vi "BRig_FPGA_v3,93__PortC.vi"() -> ()   [LabVIEW 2014]
uses:
  <vilib>/rvi/Emulation/niFpgaGetClockAttributes.vi
  <vilib>/rvi/Emulation/niFpgaSctlEmulationGetInTimedLoop.vi
  <vilib>/rvi/Emulation/niFpgaEmulationReportErrorSimple.vi
  <vilib>/rvi/eio/common/nirviEmuTemplateMethod_errors.vi
  <vilib>/rvi/Emulation/niFpgaCriticalErrorInLSC.vi
  <vilib>/eio/EIONode/EIONode.xnode
panel:
  out "fpga_solenoid_R":bool
  out "fpga_solenoid_L":bool
  out "fpga_laser2":bool
  out "fpga_laser1":bool
  in  "L2Led_ON":bool
  in  "L1Led_ON":bool
  in  "Rising(F)_or_Falling(T)":bool
  in  "Solenoid_trig_R":bool
  in  "Solenoid_trig_L":bool
  in  "Solenoid_nTotal_R":u32=100
  in  "Solenoid_nTotal_L":u32=100
  in  "L2Led_Baseline":bool
  in  "L1Led_Baseline":bool
  in  "CueLed_Baseline":bool
  in  "I_allReward":bool
  in  "AnaOut_1":i16
  in  "CueLed_Event":bool
  in  "CueLed_nValley":u32=100
  in  "CueLed_nPeak":u32=100
  in  "LC_Event_l2":bool
  in  "LC_Laser_l2":bool
  in  "LC_nShutter_l2":u32=100
  in  "LC_nValley_l2":u32=100
  in  "LC_nPeak_l2":u32=100
  in  "LR_wrong_nDelay_l2":u32
  in  "LR_reward_nDelay_l2":u32
  in  "LR_wrong_nTotal_l2":u32=100
  in  "LR_reward_nTotal_l2":u32=100
  in  "LR_wrong_laser_l2":bool
  in  "LR_wrong_Event_l2":bool
  in  "LR_reward_Laser_l2":bool
  in  "LR_reward_Event_l2":bool
  out "AnaIn_1":i16
  out "AnaIn_0":i16
  out "timeTrial_count":u32
  in  "timeTrial_trig":bool
  in  "k1__counter_per_ms":u16=100 min=100 max=40000 step=1
  in  "LC_nShutter_l1":u32=100
  in  "AnaOut_0":i16
  in  "LC_nValley_l1":u32=100
  in  "LC_nPeak_l1":u32=100
  in  "LC_Event_l1":bool
  in  "LR_wrong_nTotal_l1":u32=100
  in  "LR_wrong_nDelay_l1":u32
  in  "LR_reward_nTotal_l1":u32=100
  in  "LR_reward_nDelay_l1":u32
  in  "LR_reward_Event_l1":bool
  in  "LR_wrong_Event_l1":bool
  out "SelectWrong":bool
  out "SelectReward":bool
  in  "LR_wrong_Laser_l1":bool
  in  "LR_reward_Laser_l1":bool
  in  "Left(F)_or_Right(T)":bool
  in  "ignoreWrong":bool
  in  "SelectionState":bool
  in  "LC_Laser_l1":bool
  in  "FPGA_Stop":bool
  in  "audioTrigger_L":bool
  in  "audioTrigger_R":bool
  in  "audioFreq_L_kHz":u8=14 min=1 max=14 step=1
  in  "audioAmp_L":u16=1 min=1 max=32767 step=1
  in  "audioFreq_R_kHz":u8=14 min=1 max=14 step=1
  in  "audioAmp_R":u16=1 min=1 max=32767 step=1
  in  "A3_SL":bool
  in  "A1_SR":bool
  in  "Counts_Reset":bool
  out "A4_LickR":u32
  out "A2_LickL":u32
  in  "A6_Act":bool
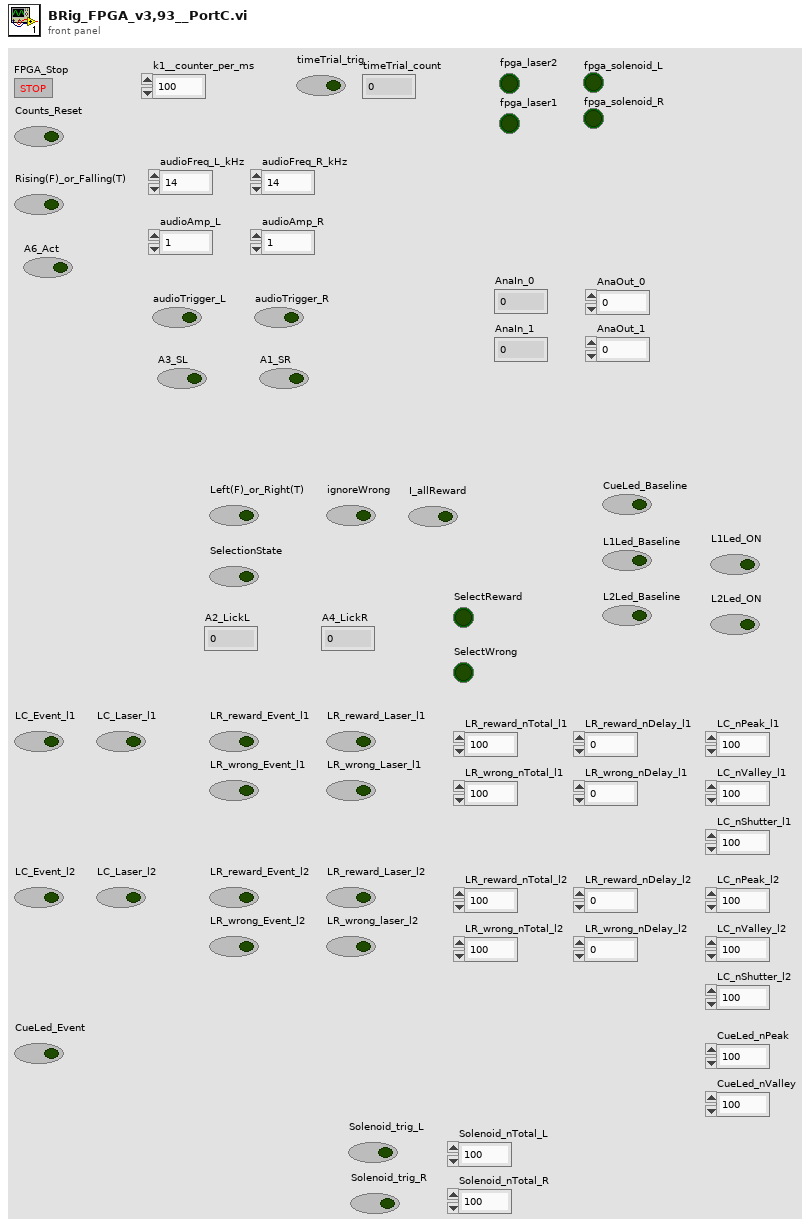
[diagram p1: front panel]
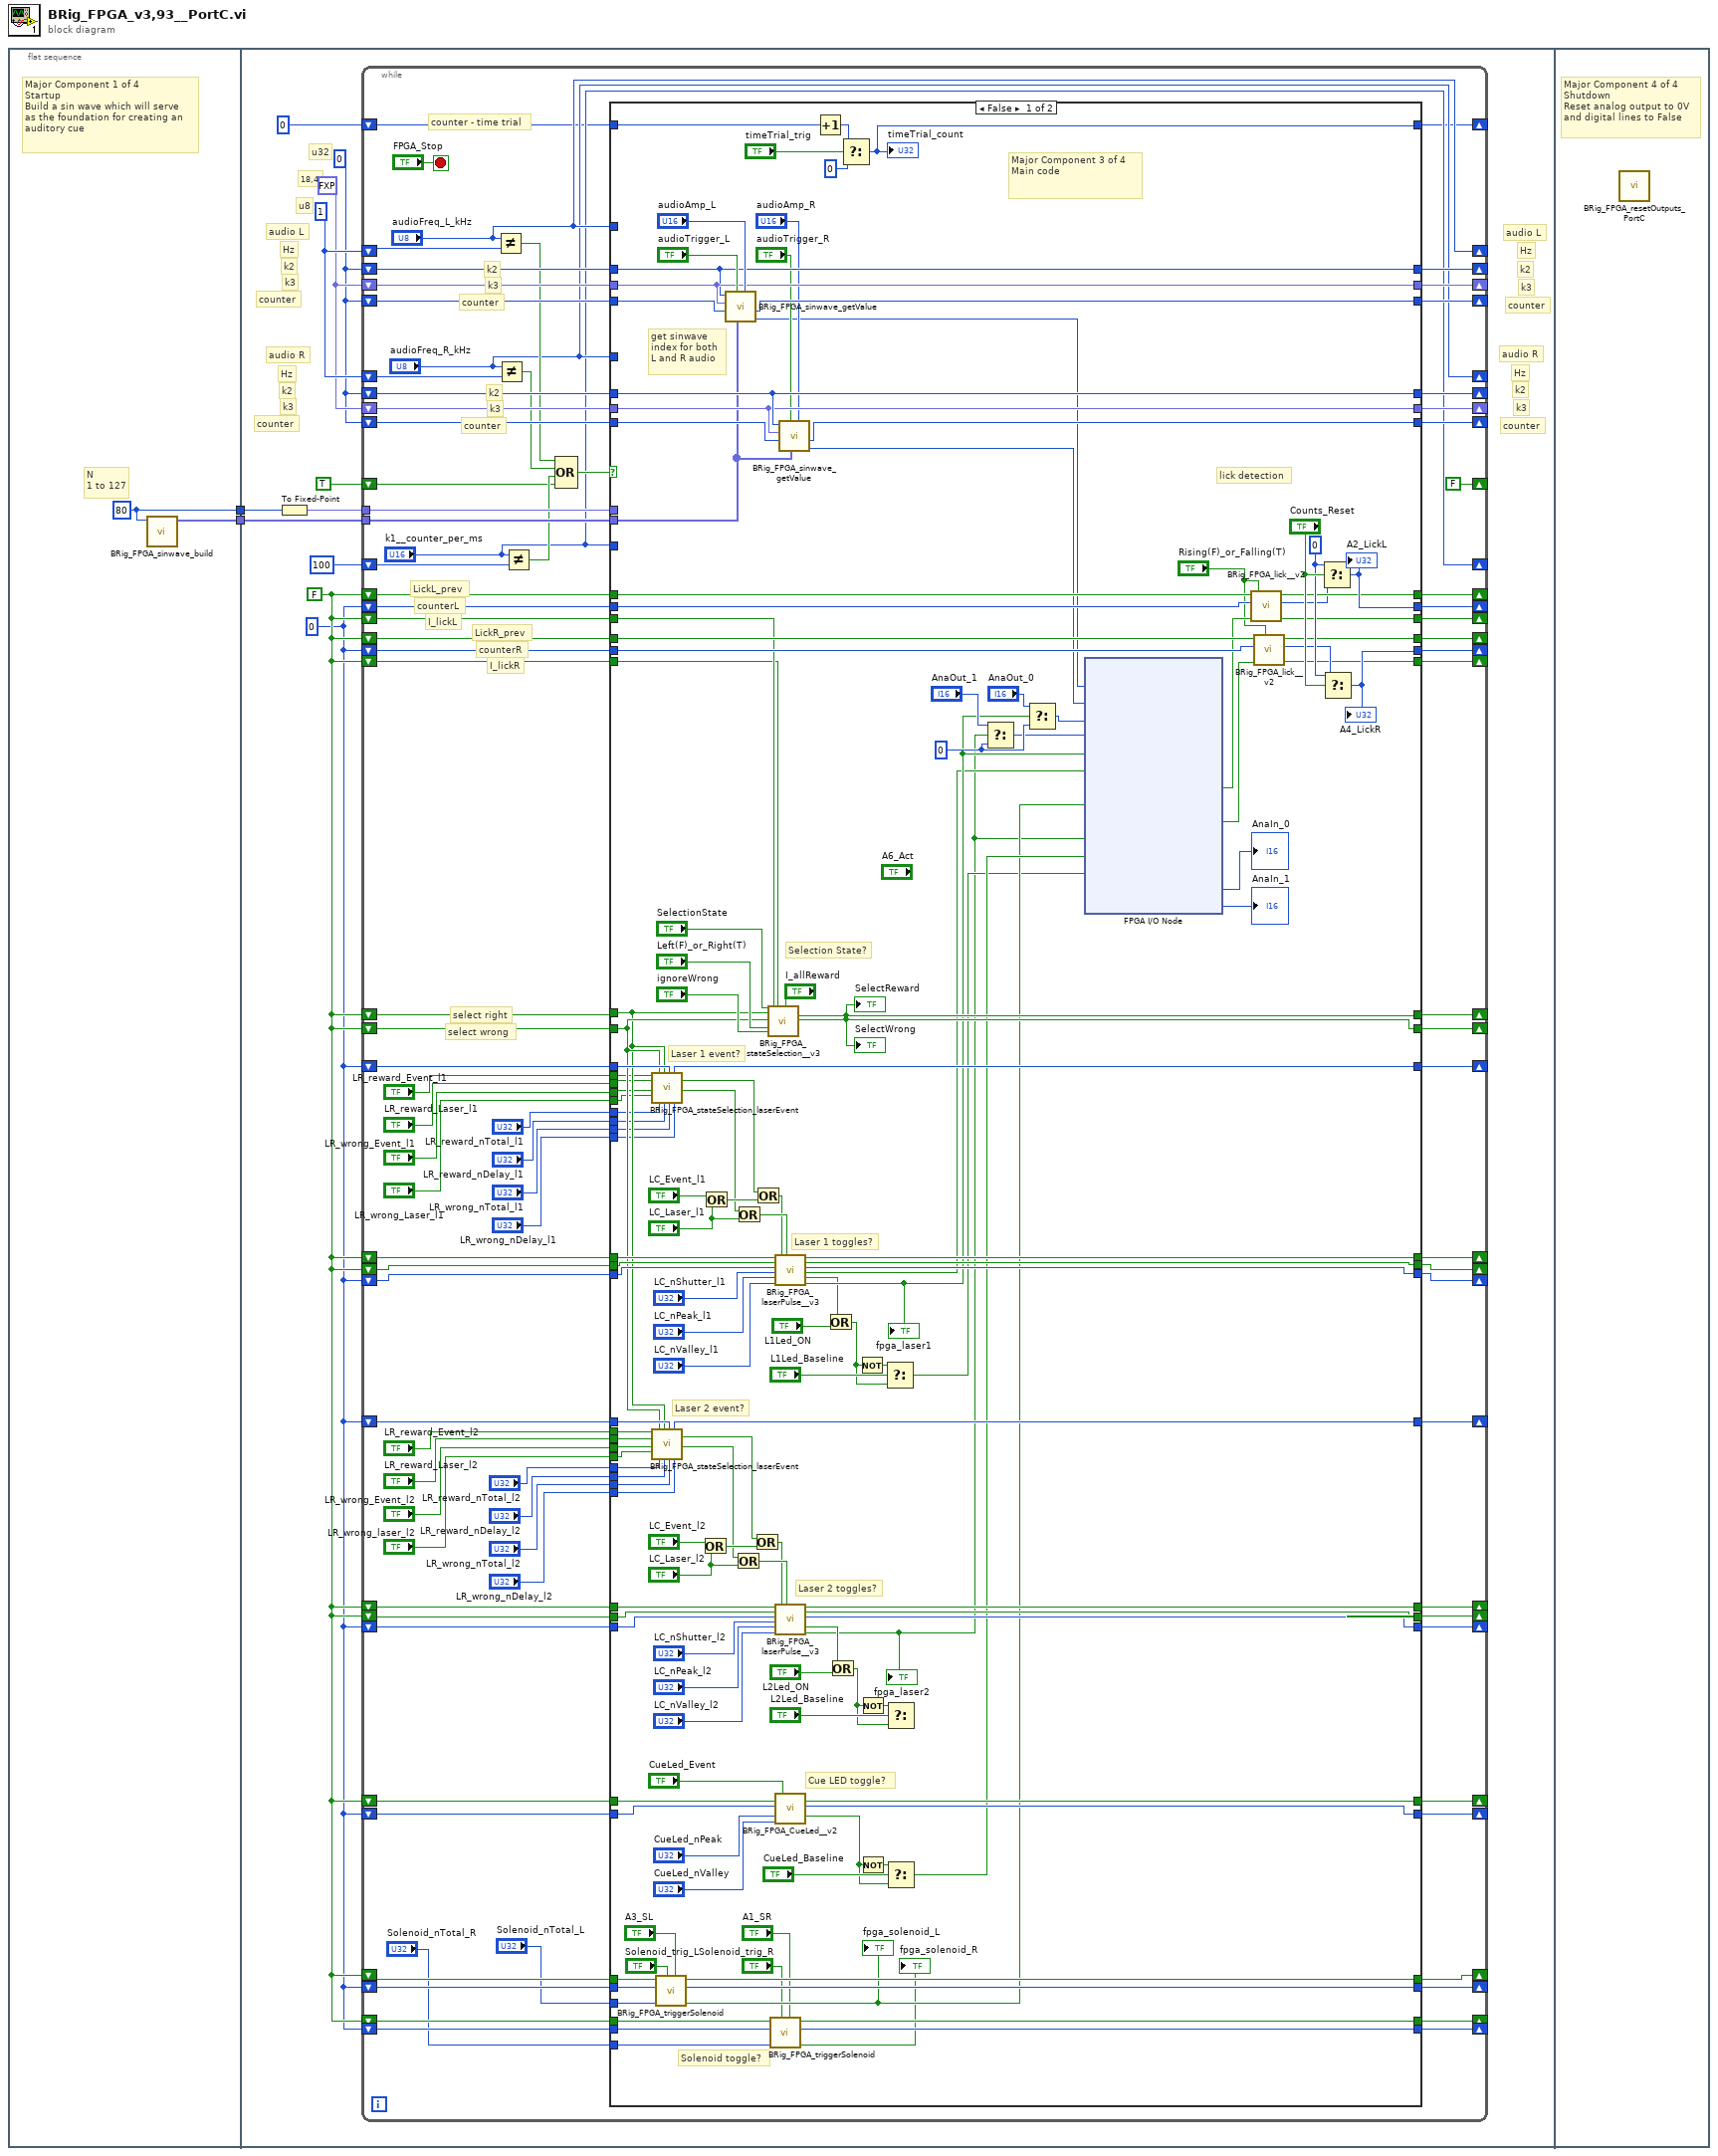
[diagram p0: block diagram]
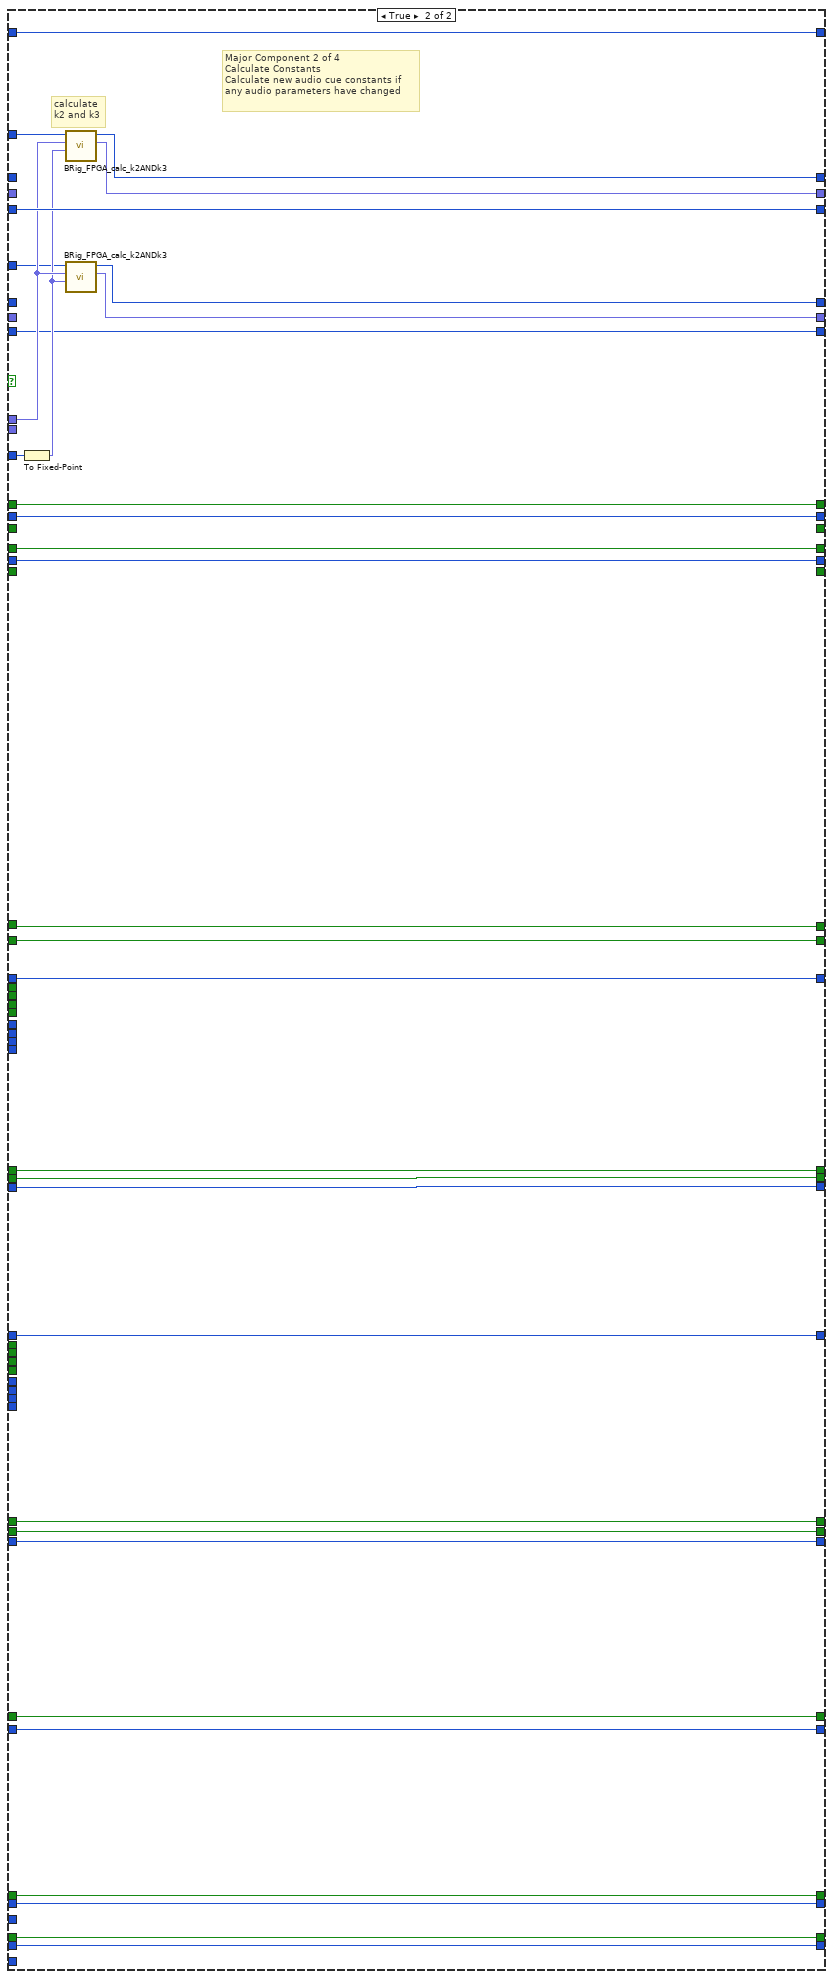
[diagram p2: hidden frame]
diagram:
  n1 = flat-sequence {
    tunnel: [w4] -> w2
    tunnel: [w3] -> w1
    tunnel: w2 -> [w15]
    tunnel: w1 -> [w14]
    frame #0 {
      w3 = 80 ("dimension size")
      # "Major Component 1 of 4\nStartup\nBuild a sin wave which will serve\nas the foundation for creating an\nauditory cue"
      # "N\n1 to 127"
      n2 = call "BRig_FPGA_sinwave_build.vi"("input_Npts"=w3) -> ("output_array_sin"=w4:fxp<+/-,16,2>[])  [unwired: 10 in]
    }
    frame #1 {
      w5 = u32 0
      w6 = FALSE
      w10 = u32 0
      w11 = fxp<+,18,4> 0.0
      w12 = u8 1
      # "counter"
      # "k3"
      # "k2"
      # "counter"
      # "k3"
      # "k2"
      # "counter"
      # "counter"
      # "u32"
      # "k3"
      # "k2"
      # "k3"
      # "18,4"
      # "u8"
      # "Hz"
      # "Hz"
      # "audio R"
      # "audio L"
      # "Hz"
      # "k2"
      # "Hz"
      # "audio R"
      # "audio L"
      n3 = To Fixed-Point(number=w14) -> (fixed-point=w13:fxp<+,7,7>)  [unwired: 1 in]
      n4 = while {
        shift-right: ["audioFreq_L_kHz"] -> _
        shift-left: w12 -> [w106]
        shift-right: [w100] -> _
        shift-left: w10 -> [w104]
        shift-right: ["audioFreq_R_kHz"] -> _
        shift-left: w12 -> [w96]
        tunnel: w15 -> [w103]
        tunnel: w13 -> [w102]
        shift-right: [w99] -> _
        shift-left: w11 -> [w101]
        shift-right: [w97] -> _
        shift-left: w10 -> [w98]
        shift-right: [w94] -> _
        shift-left: w10 -> [w95]
        shift-right: [w92] -> _
        shift-left: w11 -> [w93]
        shift-right: [w90] -> _
        shift-left: w10 -> [w91]
        shift-right: ["k1__counter_per_ms"] -> _
        shift-left: u16 100 ("y") -> [w89]
        shift-right: [FALSE] -> _
        shift-left: TRUE -> [w84]
        shift-right: [w77] -> _
        shift-left: w6 -> [w79]
        shift-right: [w76] -> _
        shift-left: w6 -> [w78]
        shift-right: [w74] -> _
        shift-left: w5 -> [w75]
        shift-right: [w72] -> _
        shift-left: w5 -> [w73]
        shift-right: [w69] -> _
        shift-left: w6 -> [w71]
        shift-right: [w68] -> _
        shift-left: w6 -> [w70]
        shift-right: [w66] -> _
        shift-left: w6 -> [w67]
        shift-right: [w64] -> _
        shift-left: w6 -> [w65]
        shift-right: [w62] -> _
        shift-left: u32 0 -> [w63]
        shift-right: [w60] -> _
        shift-left: w5 -> [w61]
        shift-right: [w59] -> _
        shift-left: w6 -> [w56]
        shift-right: [w58] -> _
        shift-left: w6 -> [w55]
        shift-right: [w57] -> _
        shift-left: w5 -> [w54]
        shift-right: [w52] -> _
        shift-left: w5 -> [w53]
        shift-right: [w51] -> _
        shift-left: w6 -> [w48]
        shift-right: [w50] -> _
        shift-left: w6 -> [w47]
        shift-right: [w49] -> _
        shift-left: w5 -> [w46]
        shift-right: [w45] -> _
        shift-left: w6 -> [w43]
        shift-right: [w44] -> _
        shift-left: w5 -> [w42]
        shift-right: [w24] -> _
        shift-left: w5 -> [w25]
        shift-right: [w21] -> _
        shift-left: w6 -> [w23]
        shift-right: [w18] -> _
        shift-left: w6 -> [w20]
        shift-right: [w17] -> _
        shift-left: w5 -> [w19]
        stop <- "FPGA_Stop" stop-if-true
        # "counter"
        # "k3"
        # "k2"
        # "counter"
        # "k3"
        # "k2"
        # "counter - time trial"
        # "I_lickR"
        # "counterR"
        # "LickR_prev"
        # "I_lickL"
        # "counterL"
        # "LickL_prev"
        # "select wrong"
        # "select right"
        n5 = Not Equal?(x="audioFreq_L_kHz", y=w106) -> (x != y?=w88:bool)
        n6 = Not Equal?(x="audioFreq_R_kHz", y=w96) -> (x != y?=w87:bool)
        n7 = Not Equal?(x="k1__counter_per_ms", y=w89) -> (x != y?=w85:bool)
        n8 = Compound Arithmetic op=OR(w88, w87, w85, w84) -> (w86:bool)
        n9 = case shown="False" w86 {
          tunnel: w104 -> [w238 _]
          tunnel: "audioFreq_L_kHz" -> [_ w284]
          tunnel: w103 -> [w231 _]
          tunnel: w102 -> [_ w280]
          tunnel: "k1__counter_per_ms" -> [_ w285]
          tunnel: w101 -> [w239 _]
          tunnel: [w238 w283] -> w100
          tunnel: [w239 w282] -> w99
          tunnel: w98 -> [w243 w281]
          tunnel: [w240 w281] -> w97
          tunnel: w95 -> [w235 _]
          tunnel: [w235 w276] -> w94
          tunnel: w93 -> [w234 _]
          tunnel: [w234 w277] -> w92
          tunnel: w91 -> [w237 w275]
          tunnel: "audioFreq_R_kHz" -> [_ w278]
          tunnel: [w236 w275] -> w90
          tunnel: w79 -> [w226 w274]
          tunnel: w78 -> [w225 w273]
          tunnel: [w230 w274] -> w77
          tunnel: [w223 w273] -> w76
          tunnel: w75 -> [w227 w272]
          tunnel: [w253 w272] -> w74
          tunnel: w73 -> [w224 w271]
          tunnel: [w250 w271] -> w72
          tunnel: w71 -> [w177 w270]
          tunnel: w70 -> [w178 w269]
          tunnel: [w197 w270] -> w69
          tunnel: [w246 w269] -> w68
          tunnel: [w216 w266] -> w59
          tunnel: [w217 w265] -> w58
          tunnel: [w218 w264] -> w57
          tunnel: w67 -> [w220 _]
          tunnel: [w229 _] -> w66
          tunnel: w65 -> [w219 _]
          tunnel: [w221 _] -> w64
          tunnel: w63 -> [w208 w268]
          tunnel: [w205 w268] -> w62
          tunnel: w61 -> [w196 w267]
          tunnel: [w195 w267] -> w60
          tunnel: w56 -> [w194 w266]
          tunnel: w55 -> [w193 w265]
          tunnel: w54 -> [w192 w264]
          tunnel: w53 -> [w180 w263]
          tunnel: [w179 w263] -> w52
          tunnel: [w175 w262] -> w51
          tunnel: [w174 w261] -> w50
          tunnel: [w173 w260] -> w49
          tunnel: w48 -> [w172 w262]
          tunnel: w47 -> [w171 w261]
          tunnel: w46 -> [w170 w260]
          tunnel: [w167 w259] -> w45
          tunnel: [w166 w258] -> w44
          tunnel: w43 -> [w165 w259]
          tunnel: w42 -> [w164 w258]
          tunnel: "LR_reward_Event_l1" -> [w148 _]
          tunnel: "LR_reward_Laser_l1" -> [w147 _]
          tunnel: "LR_wrong_Event_l1" -> [w146 _]
          tunnel: "LR_wrong_Laser_l1" -> [w145 _]
          tunnel: "LR_reward_nTotal_l1" -> [w144 _]
          tunnel: "LR_reward_nDelay_l1" -> [w143 _]
          tunnel: "LR_wrong_nTotal_l1" -> [w142 _]
          tunnel: "LR_wrong_nDelay_l1" -> [w141 _]
          tunnel: "LR_reward_Event_l2" -> [w140 _]
          tunnel: "LR_reward_Laser_l2" -> [w139 _]
          tunnel: "LR_wrong_Event_l2" -> [w138 _]
          tunnel: "LR_wrong_laser_l2" -> [w137 _]
          tunnel: "LR_reward_nTotal_l2" -> [w136 _]
          tunnel: "LR_reward_nDelay_l2" -> [w135 _]
          tunnel: "LR_wrong_nTotal_l2" -> [w134 _]
          tunnel: "LR_wrong_nDelay_l2" -> [w133 _]
          tunnel: w25 -> [w132 w257]
          tunnel: [w127 w257] -> w24
          tunnel: w23 -> [w131 w256]
          tunnel: "Solenoid_nTotal_L" -> [w130 _]
          tunnel: [w126 w256] -> w21
          tunnel: w20 -> [w122 w255]
          tunnel: w19 -> [w121 w254]
          tunnel: [w120 w255] -> w18
          tunnel: [w119 w254] -> w17
          tunnel: "Solenoid_nTotal_R" -> [w118 _]
          frame False {
            w161 = i16 0 ("f")
            w251 = u32 0 ("t")
            # "Solenoid toggle?"
            # "Cue LED toggle?"
            # "Laser 2 toggles?"
            # "Laser 2 event?"
            # "Laser 1 toggles?"
            # "Selection State?"
            # "Laser 1 event?"
            # "Major Component 3 of 4\nMain code"
            # "get sinwave\nindex for both\nL and R audio"
            # "lick detection"
            n10 = call "BRig_FPGA_stateSelection_laserEvent.vi"("I_LR_reward"=w148, "I_LR_reward_laser"=w147, "I_LR_wrong"=w146, "I_LR_wrong_laser"=w145, "I_selectWrong"=w178, "laser_reward_nTotal"=w144, "I_selectReward"=w177, "laser_reward_nDelay"=w143, "counter"=w196, "laser_wrong_nTotal"=w142, "laser_wrong_nDelay"=w141) -> ("output_counter"=w195:u32, "output_I_laserEvent"=w191:bool, "output_I_laserOn"=w190:bool)  [unwired: 6 in]
            n11 = call "BRig_FPGA_stateSelection_laserEvent.vi"("I_LR_reward"=w140, "I_LR_reward_laser"=w139, "I_LR_wrong"=w138, "I_LR_wrong_laser"=w137, "I_selectWrong"=w178, "laser_reward_nTotal"=w136, "I_selectReward"=w177, "laser_reward_nDelay"=w135, "counter"=w180, "laser_wrong_nTotal"=w134, "laser_wrong_nDelay"=w133) -> ("output_counter"=w179:u32, "output_I_laserEvent"=w176:bool, "output_I_laserOn"=w181:bool)  [unwired: 6 in]
            n12 = call "BRig_FPGA_triggerSolenoid.vi"("input_Solenoid_MTrig"="A3_SL", "input_Solenoid_trig"="Solenoid_trig_L", "input_threshold"=w130, "input_counter"=w132, "input_trig"=w131) -> ("output_Solenoid_OnOff"=w125:bool, "output_counter"=w127:u32, "output_trig"=w126:bool)  [unwired: 4 in]
            "fpga_solenoid_L" <- w125
            n13 = Or(x="LC_Event_l2", y="LC_Laser_l2") -> (x .or. y?=w185:bool)
            n14 = Or(x="LC_Event_l1", y="LC_Laser_l1") -> (x .or. y?=w212:bool)
            n15 = call "BRig_FPGA_sinwave_getValue.vi"("audioAmp"="audioAmp_L", "sinwave"=w231, "audioTrigger"="audioTrigger_L", "counter"=w243, "k3"=w239, "k2"=w238) -> ("output_audioValue"=w203:i16, "output_counter"=w240:u32)  [unwired: 4 in]
            n16 = Or(x=w181, y="LC_Laser_l2") -> (x .or. y?=w183:bool)
            n17 = Or(x=w190, y="LC_Laser_l1") -> (x .or. y?=w210:bool)
            n18 = Or(x=w176, y=w185) -> (x .or. y?=w182:bool)
            n19 = Or(x=w191, y=w212) -> (x .or. y?=w209:bool)
            n20 = call "BRig_FPGA_stateSelection__v3.vi"("I_selectionState"="SelectionState", "I_selectRight"=w177, "I_selectWrong"=w178, "I_Left(F)_or_Right(T)"="Left(F)_or_Right(T)", "I_ignoreWrong"="ignoreWrong", "I_lickL"=w220, "I_lickR"=w219, "I_allReward"="I_allReward") -> ("output__I_selectRight"=w197:bool, "output__I_selectWrong"=w246:bool)  [unwired: 18 in]
            "SelectWrong" <- w246
            "SelectReward" <- w197
            n21 = call "BRig_FPGA_triggerSolenoid.vi"("input_Solenoid_MTrig"="A1_SR", "input_Solenoid_trig"="Solenoid_trig_R", "input_threshold"=w118, "input_counter"=w121, "input_trig"=w122) -> ("output_Solenoid_OnOff"=→"fpga_solenoid_R":bool, "output_counter"=w119:u32, "output_trig"=w120:bool)  [unwired: 4 in]
            n22 = call "BRig_FPGA_laserPulse__v3.vi"("I_shutter"=w194, "I_peak"=w193, "count"=w192, "laser_Nshutter"="LC_nShutter_l1", "laser_Npeak"="LC_nPeak_l1", "laser_Nvalley"="LC_nValley_l1", "I_laserEvent"=w209, "I_laser"=w210) -> ("output_I_shutter"=w216:bool, "output_I_peak"=w217:bool, "output_count"=w218:u32, "output_shutter"=w109:bool, "output_led"=w114:bool, "output_laser"=w159:bool)  [unwired: 6 in]
            "fpga_laser1" <- w159
            n23 = call "BRig_FPGA_laserPulse__v3.vi"("I_shutter"=w172, "I_peak"=w171, "count"=w170, "laser_Nshutter"="LC_nShutter_l2", "laser_Npeak"="LC_nPeak_l2", "laser_Nvalley"="LC_nValley_l2", "I_laserEvent"=w182, "I_laser"=w183) -> ("output_I_shutter"=w175:bool, "output_I_peak"=w174:bool, "output_count"=w173:u32, "output_led"=w111:bool, "output_laser"=w108:bool)  [unwired: 6 in, 1 out]
            "fpga_laser2" <- w108
            n24 = call "BRig_FPGA_CueLed__v2.vi"("I_peak"=w165, "count"=w164, "laser_Npeak"="CueLed_nPeak", "laser_Nvalley"="CueLed_nValley", "I_CueLed_Event"="CueLed_Event") -> ("output_I_peak"=w167:bool, "output_count"=w166:u32, "output_led"=w153:bool)  [unwired: 12 in]
            n25 = call "BRig_FPGA_sinwave_getValue.vi"("audioAmp"="audioAmp_R", "sinwave"=w231, "audioTrigger"="audioTrigger_R", "counter"=w237, "k3"=w234, "k2"=w235) -> ("output_audioValue"=w202:i16, "output_counter"=w236:u32)  [unwired: 4 in]
            n26 = Increment(x=w208) -> (x+1=w207:u32)
            n27 = Or(x=w114, y="L1Led_ON") -> (x .or. y?=w113:bool)
            n28 = Or(x=w111, y="L2Led_ON") -> (x .or. y?=w110:bool)
            n29 = Select(t=w207, s="timeTrial_trig", f=u32 0) -> (s? t:f=w205:u32)
            "timeTrial_count" <- w205
            n30 = Not(x=w113) -> (.not. x?=w152:bool)
            n31 = Not(x=w110) -> (.not. x?=w150:bool)
            n32 = Not(x=w153) -> (.not. x?=w155:bool)
            n33 = Select(t=w152, s="L1Led_Baseline", f=w113) -> (s? t:f=w116:bool)
            n34 = Select(t=w150, s="L2Led_Baseline", f=w110) -> ()  [unwired: 1 out]
            n35 = Select(t=w155, s="CueLed_Baseline", f=w153) -> (s? t:f=w156:bool)
            n36 = Select(t="AnaOut_1", s=w108, f=w161) -> (s? t:f=w158:i16)
            n37 = Select(t="AnaOut_0", s=w159, f=w161) -> (s? t:f=w162:i16)
            n38 = xnode "FPGA I/O Node"("AudioOut/Left"=w203, "AudioOut/Right"=w202, "ConnectorC/AO0"=w162, "ConnectorC/AO1"=w158, "ConnectorC/DIO0"=w159, "ConnectorC/DIO1"=w109, "ConnectorC/DIO3"=w125, "ConnectorC/DIO5"=w108, "ConnectorC/DIO6"=w156, "ConnectorC/DIO7"=w116) -> ("ConnectorC/DIO2"=w201:bool, "ConnectorC/DIO4"=w200:bool, "ConnectorC/AI0"=→"AnaIn_0":i16, "ConnectorC/AI1"=→"AnaIn_1":i16)  [unwired: 14 in, 14 out]
            n39 = call "BRig_FPGA_lick__v2.vi"("Rising(F)_or_Falling(T)"="Rising(F)_or_Falling(T)", "I_stateDetector_new"=w201, "counter"=w227, "I_stateDetector_prev"=w226) -> ("output_I_lick"=w229:bool, "output_counter"=w228:u32, "output_I_stateDetector_prev"=w230:bool)  [unwired: 5 in]
            n40 = call "BRig_FPGA_lick__v2.vi"("Rising(F)_or_Falling(T)"="Rising(F)_or_Falling(T)", "I_stateDetector_new"=w200, "counter"=w224, "I_stateDetector_prev"=w225) -> ("output_I_lick"=w221:bool, "output_counter"=w222:u32, "output_I_stateDetector_prev"=w223:bool)  [unwired: 5 in]
            n41 = Select(t=w251, s="Counts_Reset", f=w228) -> (s? t:f=w253:u32)
            "A2_LickL" <- w253
            n42 = Select(t=w251, s="Counts_Reset", f=w222) -> (s? t:f=w250:u32)
            "A4_LickR" <- w250
          }
          frame True {
            # "Major Component 2 of 4\nCalculate Constants\nCalculate new audio cue constants if\nany audio parameters have changed"
            # "calculate\nk2 and k3"
            n43 = To Fixed-Point(number=w285) -> (fixed-point=w279:fxp<+,16,16>)  [unwired: 1 in]
            n44 = call "BRig_FPGA_calc_k2ANDk3.vi"("input_k1[count/ms]"=w279, "input_Npts"=w280, "input_freq[kHz]"=w284) -> ("output_k3"=w282:fxp<+,18,4>, "output_k2"=w283:u32)  [unwired: 7 in]
            n45 = call "BRig_FPGA_calc_k2ANDk3.vi"("input_k1[count/ms]"=w279, "input_Npts"=w280, "input_freq[kHz]"=w278) -> ("output_k3"=w277:fxp<+,18,4>, "output_k2"=w276:u32)  [unwired: 7 in]
          }
        }
      }
    }
    frame #2 {
      # "Major Component 4 of 4\nShutdown\nReset analog output to 0V\nand digital lines to False"
      n46 = call "BRig_FPGA_resetOutputs_PortC.vi"() -> ()  [unwired: 12 in]
    }
  }
